vi "constant vi validation Args.vi"(11 "Constant Argument Window":refnum<vi>) -> (3 "Proceed with Scripting":bool)   [LabVIEW 2020, in "Panther Dashboard.lvlib"]
uses:
  Panther Dashboard.lvlib
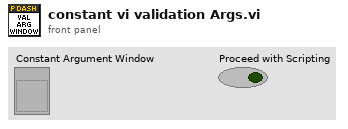
[diagram p1: front panel]
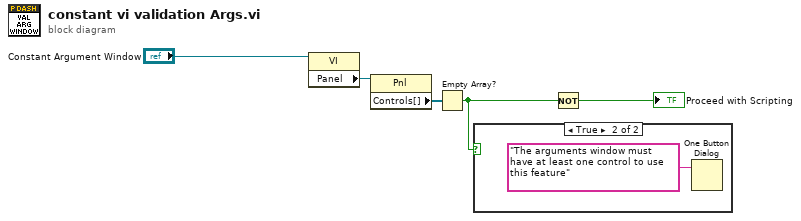
[diagram p0: block diagram]
diagram:
  n1 = property class="VI"(reference="Constant Argument Window") -> ("Panel"=w4:refnum<vi>)  [unwired: 1 in, 2 out]
  n2 = property class="Pnl"(reference=w4) -> ("Controls[]"=w3:refnum<vi>[])  [unwired: 1 in, 2 out]
  n3 = Empty Array?(array=w3) -> (empty?=w2:bool)
  n4 = case shown="True" w2 {
    frame False {
    }
    frame True {
      n5 = One Button Dialog(message="The arguments window must have at least one control to use this feature" ("format string")) -> ()  [unwired: 1 in, 1 out]
    }
  }
  n6 = Not(x=w2) -> (.not. x?=→"Proceed with Scripting":bool)
